vi "AB_900_1000_Project_RESTfulWebService_Info.vi"(7 "action":T2, 8 "error in (no error)":errorcluster, 10 "RESTfulWebServiceInfo in":T1, 11 "Object In":T3) -> (0 "error out":errorcluster, 2 "RESTfulWebServiceInfo out":T1, 3 "Object Out":T3)   [LabVIEW 2020]
uses:
  <resource>/Framework/Providers/API/ItemRef.ctl
  <vilib>/AppBuilder/RW_Project/AB_RW_Project_PropBag_Action.ctl
  <vilib>/AppBuilder/RW_Project/AB_RW_Project_RESTful_RoutingTemplate.ctl
  <vilib>/AppBuilder/AB_Classes/RESTful/AB_RESTful_RoutingType.ctl
  <vilib>/AppBuilder/AB_Classes/RESTful/AB_RESTful_HTTPMethodType.ctl
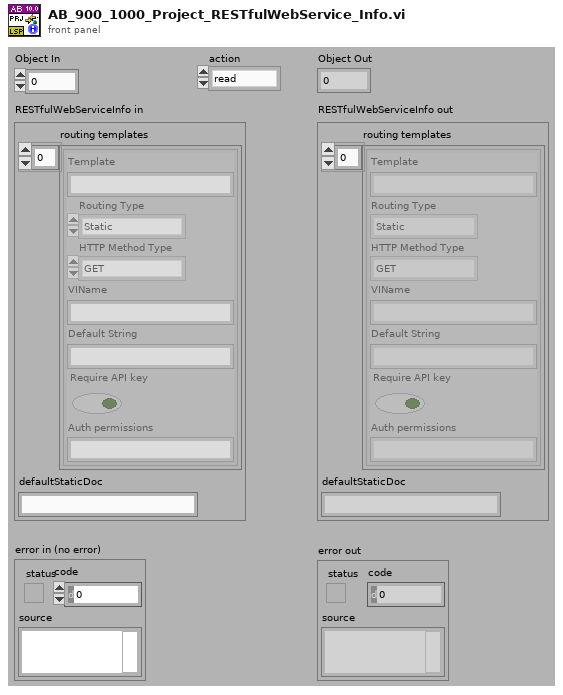
[diagram p1: front panel]
types:
  T1 = cluster{"routing templates":cluster{"Template":string, "Routing Type":enum32{"Method", "Static"}, "HTTP Method Type":enum32{"GET", "POST", "PUT", "DELETE"}, "VIName":string, "Default String":string, "Require API key":bool, "Auth permissions":string}[], "defaultStaticDoc":string}
  T2 = typedef "AB_RW_Project_PropBag_Action.ctl" = enum16{"read", "write", "clear", "readPrevious", "writePrevious", "clearPrevious"}
  T3 = typedef "ItemRef.ctl" = u64
  T4 = typedef "AB_RW_Project_RESTful_RoutingTemplate.ctl" = cluster{"Template":string, "Routing Type":T5, "HTTP Method Type":T6, "VIName":string, "Default String":string, "Require API key":bool, "Auth permissions":string}
  T5 = typedef "AB_RESTful_RoutingType.ctl" = enum32{"Method", "Static"}
  T6 = typedef "AB_RESTful_HTTPMethodType.ctl" = enum32{"GET", "POST", "PUT", "DELETE"}
  T7 = cluster{"Template":string, "Routing Type":enum32{"Method", "Static"}, "HTTP Method Type":enum32{"GET", "POST", "PUT", "DELETE"}, "VIName":string, "Default String":string, "Require API key":bool, "Auth permissions":string}[]
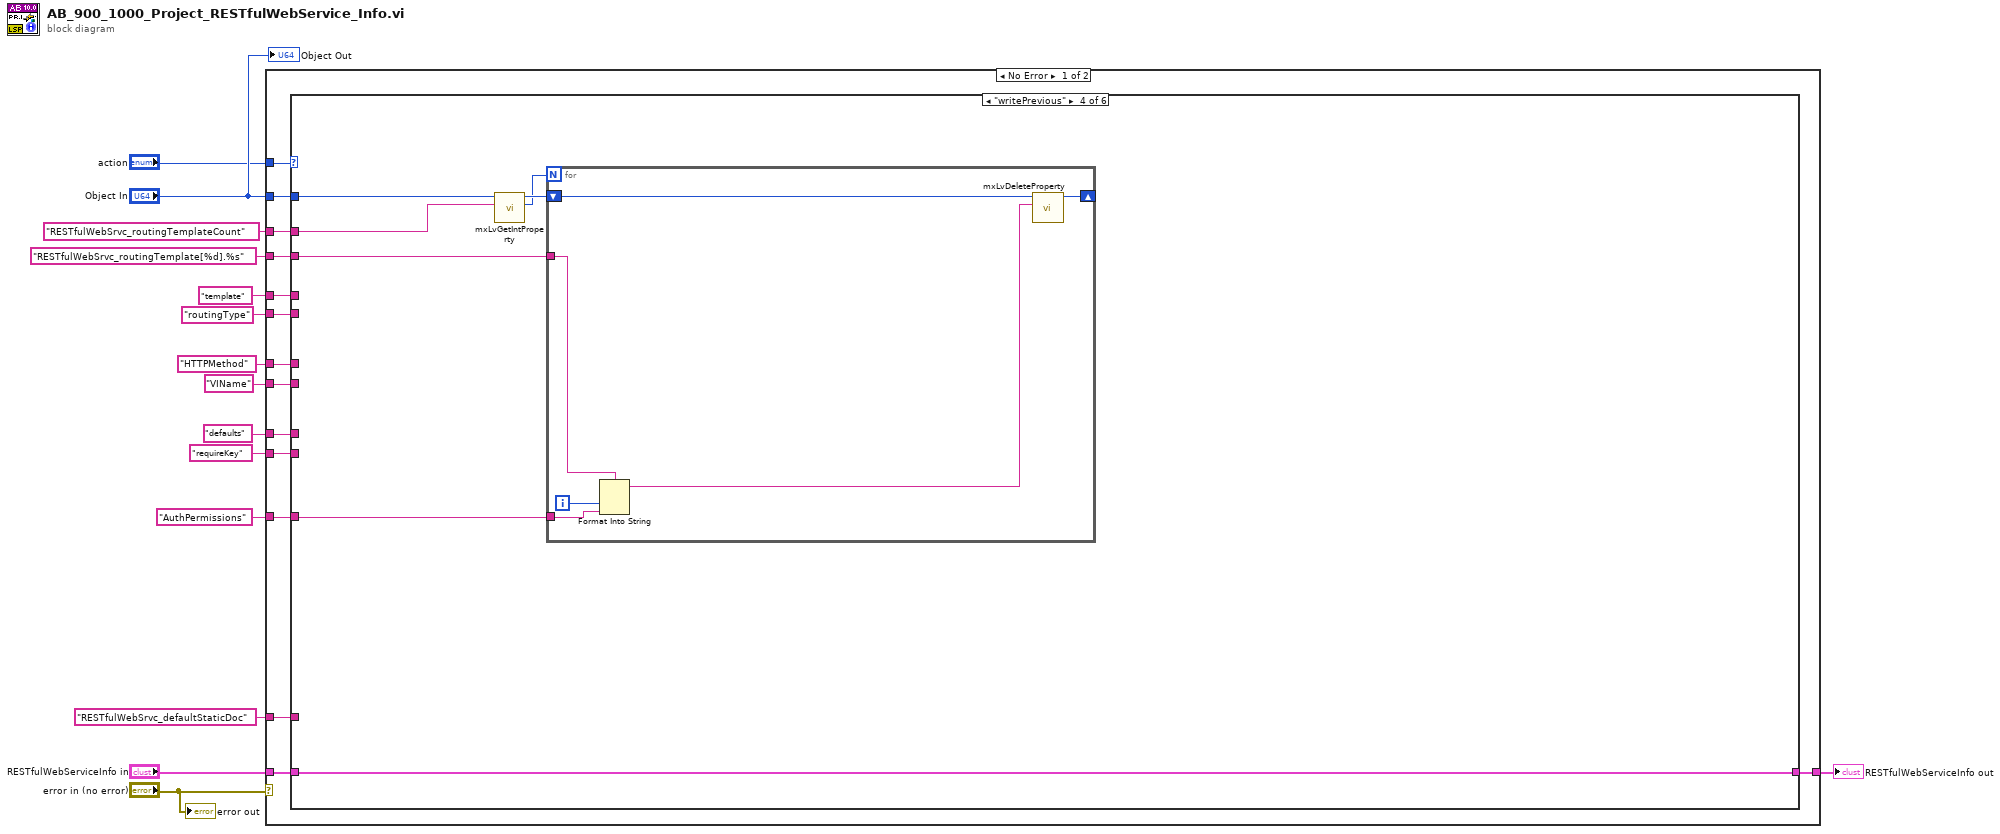
[diagram p0: block diagram]
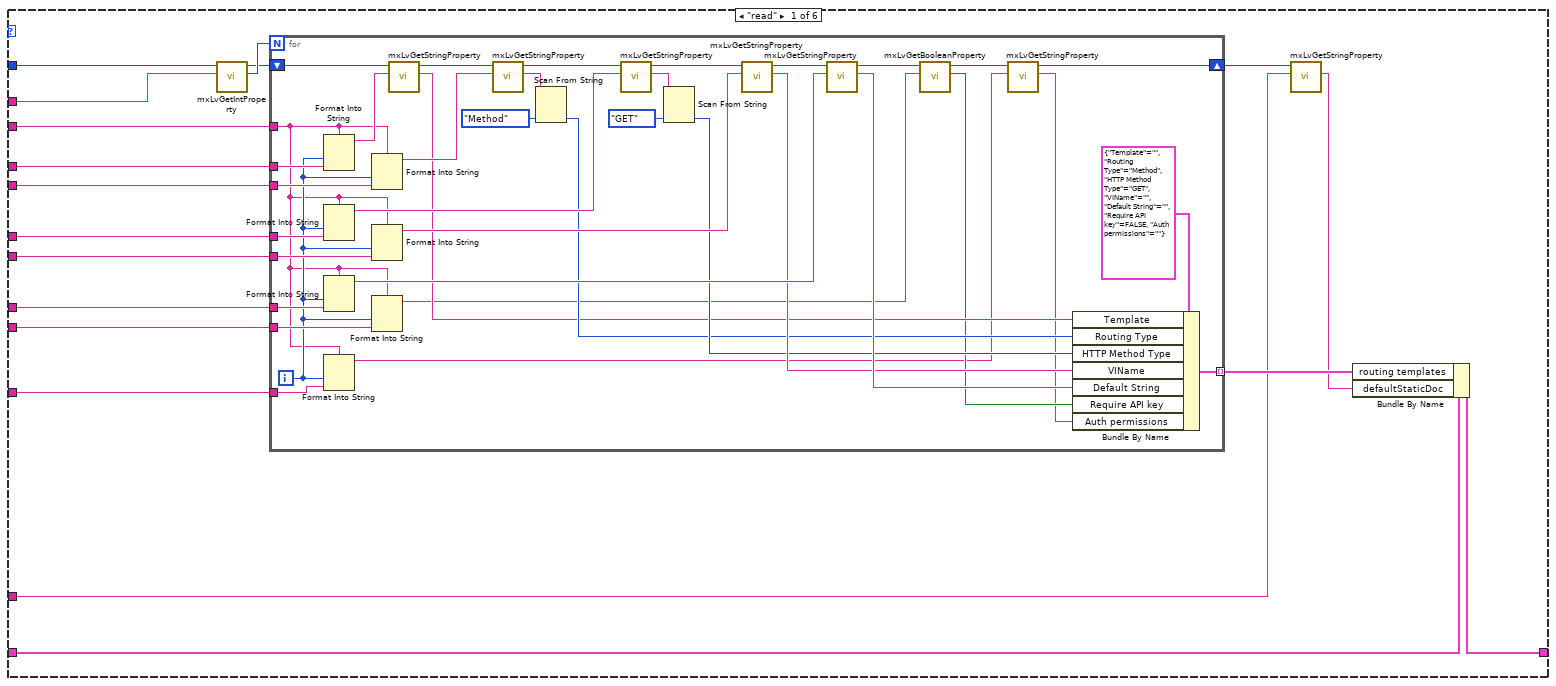
[diagram p2: hidden frame]
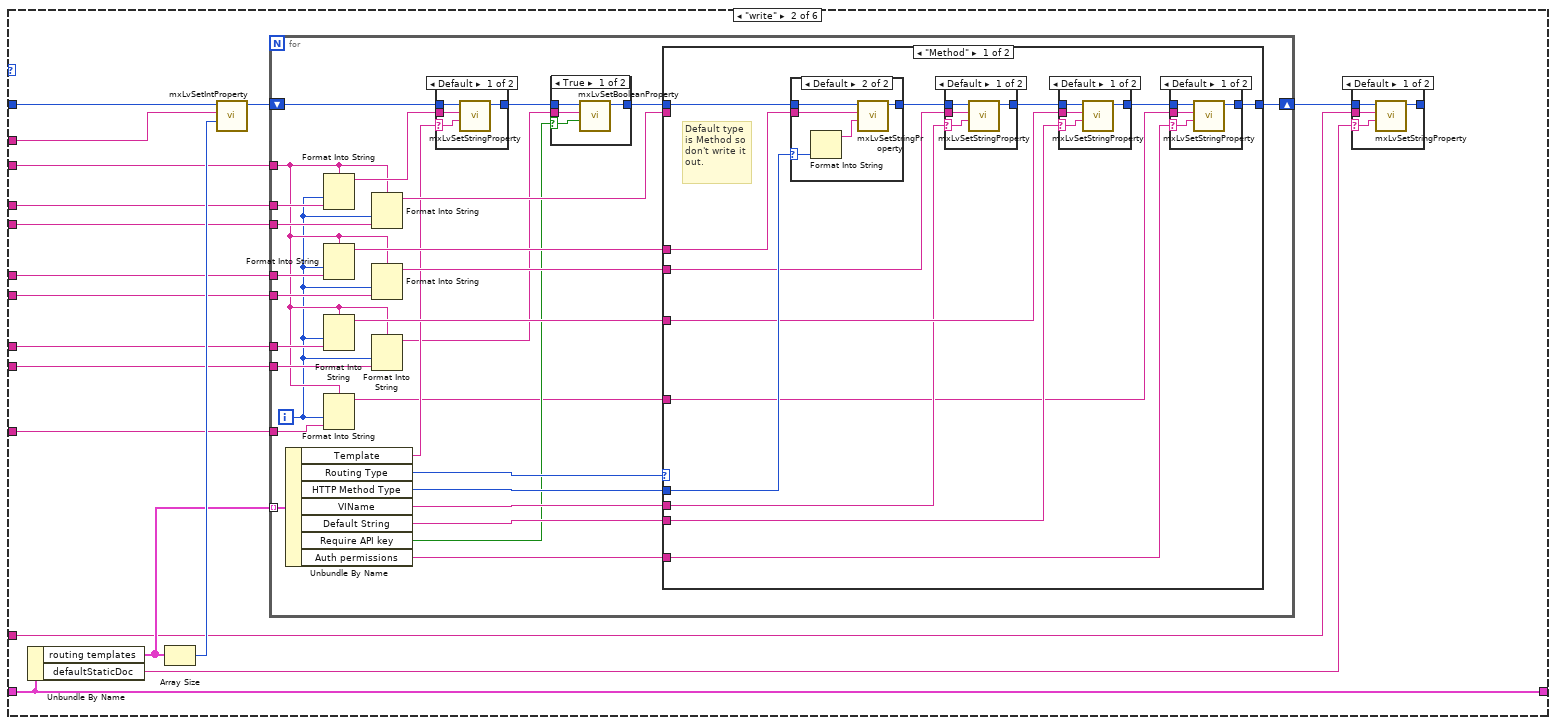
[diagram p3: hidden frame]
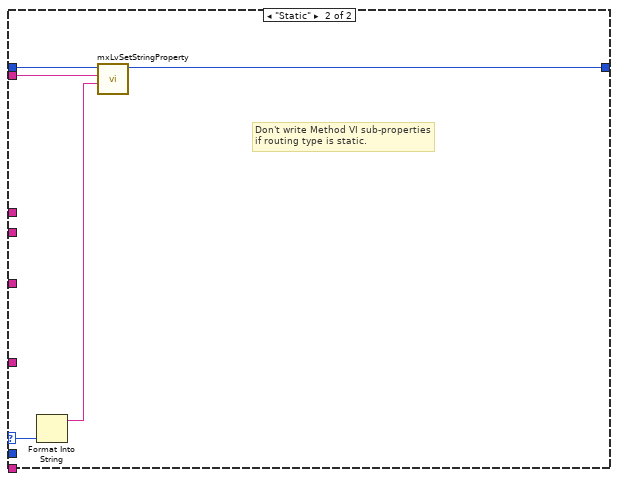
[diagram p10: hidden frame]
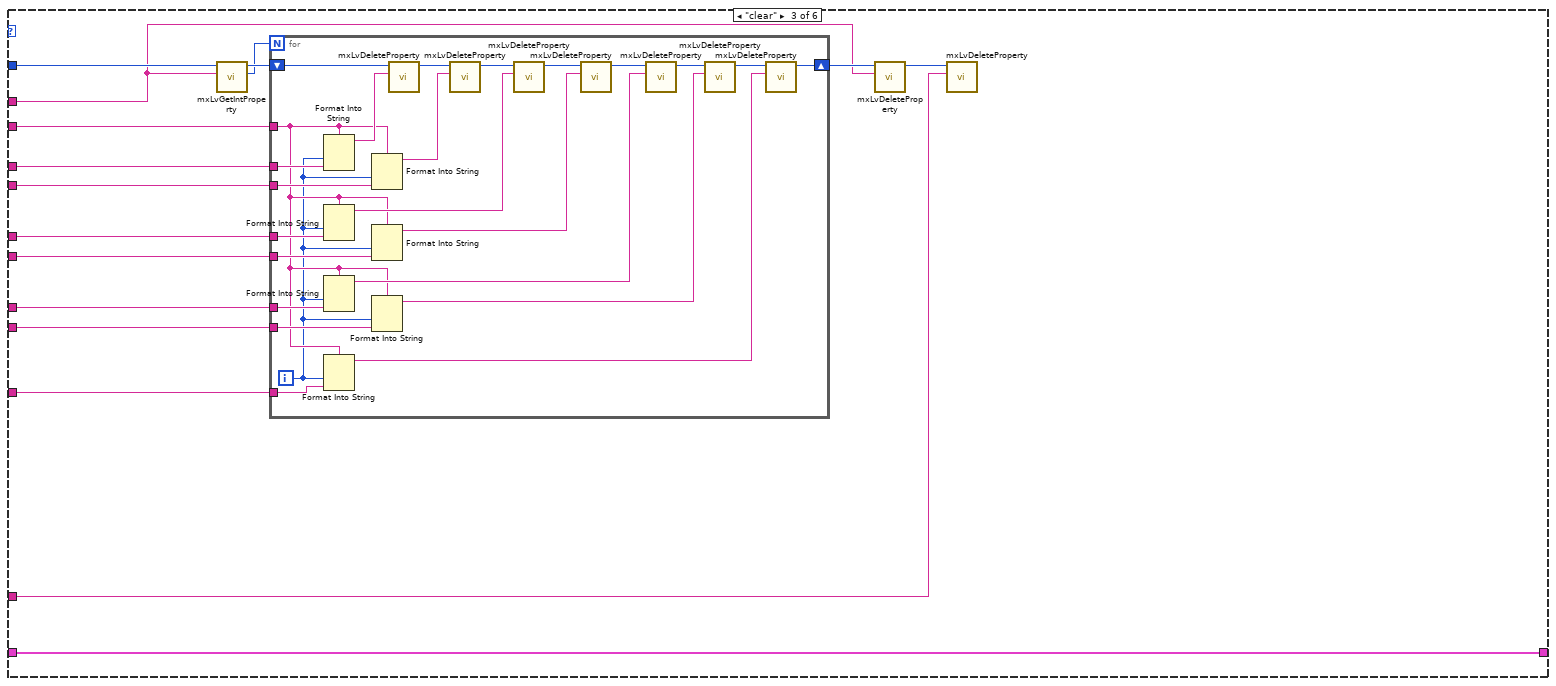
[diagram p12: hidden frame]
diagram:
  n1 = case shown="No Error" "error in (no error)" {
    tunnel: "Object In" -> [w29 _]
    tunnel: [w23 _] -> w8
    tunnel: "RESTfulWebSrvc_routingTemplateCount" ("Tag") -> [w28 _]
    tunnel: "RESTfulWebSrvc_routingTemplate[%d].%s" ("Tag") -> [w27 _]
    tunnel: "template" ("Tag") -> [w26 _]
    tunnel: "RESTfulWebServiceInfo in" -> [w25 _]
    tunnel: "action" -> [w24 _]
    tunnel: "routingType" ("Tag") -> [w22 _]
    tunnel: "HTTPMethod" ("Tag") -> [w21 _]
    tunnel: "VIName" ("Tag") -> [w20 _]
    tunnel: "defaults" ("Tag") -> [w19 _]
    tunnel: "requireKey" ("Tag") -> [w18 _]
    tunnel: "RESTfulWebSrvc_defaultStaticDoc" ("Tag") -> [w17 _]
    tunnel: "AuthPermissions" ("Tag") -> [w16 _]
    frame No Error {
      n2 = case shown="\"writePrevious\"" w24 {
        tunnel: w29 -> [w41 w98 w198 w229 _ _]
        tunnel: w28 -> [w47 w100 w189 w226 _ _]
        tunnel: w27 -> [w45 w96 w196 w227 _ _]
        tunnel: w26 -> [w40 w95 w195 _ _ _]
        tunnel: w25 -> [w42 w99 w197 w228 w237 w238]
        tunnel: [w43 w99 w197 w228 w237 w238] -> w23
        tunnel: w22 -> [w39 w94 w194 _ _ _]
        tunnel: w21 -> [w38 w93 w193 _ _ _]
        tunnel: w20 -> [w37 w92 w192 _ _ _]
        tunnel: w19 -> [w36 w91 w191 _ _ _]
        tunnel: w18 -> [w34 w89 w188 _ _ _]
        tunnel: w17 -> [w32 w87 w185 _ _ _]
        tunnel: w16 -> [w30 w85 w184 w224 _ _]
        frame "read" {
          n3 = call <resource>:"mxLvGetIntProperty.vi"("Tag"=w47, "Item"=w41) -> ("Value"=w46:i32, "Item"=w44:T3)  [unwired: 1 in, 7 out]
          n4 = for {
            N: w46 -> [_]
            shift-right: [w50] -> w33
            shift-left: w44 -> [w84]
            tunnel: w45 -> [w53]
            tunnel: w40 -> [w81]
            tunnel: w39 -> [w80]
            tunnel: w38 -> [w79]
            tunnel: w37 -> [w78]
            tunnel: w36 -> [w77]
            tunnel: [w60] -> w35 mode=indexing
            tunnel: w34 -> [w57]
            tunnel: w30 -> [w52]
            i -> [w54]
            n5 = Format Into String(format string=w53, w54, w81) -> (resulting string=w76:string)  [unwired: 2 in, 1 out]
            n6 = Format Into String(format string=w53, w54, w79) -> (resulting string=w71:string)  [unwired: 2 in, 1 out]
            n7 = Format Into String(format string=w53, w54, w77) -> (resulting string=w66:string)  [unwired: 2 in, 1 out]
            n8 = Format Into String(format string=w53, w54, w52) -> (resulting string=w48:string)  [unwired: 2 in, 1 out]
            n9 = Format Into String(format string=w53, w54, w80) -> (resulting string=w75:string)  [unwired: 2 in, 1 out]
            n10 = Format Into String(format string=w53, w54, w78) -> (resulting string=w67:string)  [unwired: 2 in, 1 out]
            n11 = Format Into String(format string=w53, w54, w57) -> (resulting string=w56:string)  [unwired: 2 in, 1 out]
            n12 = call <resource>:"mxLvGetStringProperty.vi"("Tag"=w76, "Item"=w84) -> ("Value"=w61:string, "Item"=w83:T3)  [unwired: 1 in, 7 out]
            n13 = call <resource>:"mxLvGetStringProperty.vi"("Tag"=w75, "Item"=w83) -> ("Value"=w82:string, "Item"=w72:T3)  [unwired: 1 in, 7 out]
            n14 = Scan From String(input string=w82, default 1=AB_RESTful_RoutingType."Method" ("Routing Type")) -> (output 1=w62:T5)  [unwired: 3 in, 3 out]
            n15 = call <resource>:"mxLvGetStringProperty.vi"("Tag"=w71, "Item"=w72) -> ("Value"=w73:string, "Item"=w68:T3)  [unwired: 1 in, 7 out]
            n16 = Scan From String(input string=w73, default 1=AB_RESTful_HTTPMethodType."GET" ("HTTP Method Type")) -> (output 1=w63:T6)  [unwired: 3 in, 3 out]
            n17 = call <resource>:"mxLvGetStringProperty.vi"("Tag"=w67, "Item"=w68) -> ("Value"=w64:string, "Item"=w69:T3)  [unwired: 1 in, 7 out]
            n18 = call <resource>:"mxLvGetStringProperty.vi"("Tag"=w66, "Item"=w69) -> ("Value"=w65:string, "Item"=w59:T3)  [unwired: 1 in, 7 out]
            n19 = call <resource>:"mxLvGetBooleanProperty.vi"("Tag"=w56, "Item"=w59) -> ("Value"=w58:bool, "Item"=w51:T3)  [unwired: 1 in, 7 out]
            n20 = call <resource>:"mxLvGetStringProperty.vi"("Tag"=w48, "Item"=w51) -> ("Value"=w49:string, "Item"=w50:T3)  [unwired: 1 in, 7 out]
            n21 = Bundle By Name(cluster=T4 {"Template"="", "Routing Type"=enum."Method", "HTTP Method Type"=enum."GET", "VIName"="", "Default String"="", "Require API key"=FALSE, "Auth permissions"=""} ("RESTful VI routing template"), "Template"=w61, "Routing Type"=w62, "HTTP Method Type"=w63, "VIName"=w64, "Default String"=w65, "Require API key"=w58, "Auth permissions"=w49) -> (w60:T4)
          }
          n22 = call <resource>:"mxLvGetStringProperty.vi"("Tag"=w32, "Item"=w33) -> ("Value"=w31:string)  [unwired: 1 in, 8 out]
          n23 = Bundle By Name(cluster=w42, "routing templates"=w35, "defaultStaticDoc"=w31) -> (w43:T1)
        }
        frame "write" {
          n24 = Unbundle By Name(w99) -> ("routing templates"=w90:T7, "defaultStaticDoc"=w86:string)
          n25 = Array Size(array=w90) -> (size(s)=w101:i32)
          n26 = call <resource>:"mxLvSetIntProperty.vi"("Value (0)"=w101, "Tag"=w100, "Item"=w98) -> ("Item"=w97:T3)  [unwired: 2 in, 6 out]
          n27 = for {
            shift-right: [w121] -> w88
            shift-left: w97 -> [w118]
            tunnel: w96 -> [w111]
            tunnel: w95 -> [w134]
            tunnel: w94 -> [w133]
            tunnel: w93 -> [w132]
            tunnel: w92 -> [w131]
            tunnel: w91 -> [w130]
            tunnel: w90 -> [w126] mode=indexing
            tunnel: w89 -> [w116]
            tunnel: w85 -> [w109]
            i -> [w110]
            n28 = Unbundle By Name(w126) -> ("Template"=w120:string, "Routing Type"=w117:enum32{"Method", "Static"}, "HTTP Method Type"=w125:enum32{"GET", "POST", "PUT", "DELETE"}, "VIName"=w124:string, "Default String"=w123:string, "Require API key"=w113:bool, "Auth permissions"=w107:string)
            n29 = Format Into String(format string=w111, w110, w134) -> (resulting string=w119:string)  [unwired: 2 in, 1 out]
            n30 = Format Into String(format string=w111, w110, w132) -> (resulting string=w128:string)  [unwired: 2 in, 1 out]
            n31 = Format Into String(format string=w111, w110, w130) -> (resulting string=w122:string)  [unwired: 2 in, 1 out]
            n32 = Format Into String(format string=w111, w110, w109) -> (resulting string=w108:string)  [unwired: 2 in, 1 out]
            n33 = Format Into String(format string=w111, w110, w133) -> (resulting string=w129:string)  [unwired: 2 in, 1 out]
            n34 = Format Into String(format string=w111, w110, w131) -> (resulting string=w127:string)  [unwired: 2 in, 1 out]
            n35 = Format Into String(format string=w111, w110, w116) -> (resulting string=w112:string)  [unwired: 2 in, 1 out]
            n36 = case shown="Default" w120 {
              selector: w120 -> [w179 _]
              tunnel: w118 -> [w182 w183]
              tunnel: w119 -> [w181 _]
              tunnel: [w180 w183] -> w115
              frame Default {
                n37 = call <resource>:"mxLvSetStringProperty.vi"("Value (\"\")"=w179, "Tag"=w181, "Item"=w182) -> ("Item"=w180:T3)  [unwired: 2 in, 6 out]
              }
              frame "" {
              }
            }
            n38 = case shown="True" w113 {
              selector: w113 -> [w137 _]
              tunnel: w115 -> [w138 w139]
              tunnel: w112 -> [w135 _]
              tunnel: [w136 w139] -> w114
              frame True {
                n39 = call <resource>:"mxLvSetBooleanProperty.vi"("Value (F)"=w137, "Tag"=w135, "Item"=w138) -> ("Item"=w136:T3)  [unwired: 2 in, 6 out]
              }
              frame False {
              }
            }
            n40 = case shown="\"Method\"" w117 {
              selector: w117 -> [_ w174]
              tunnel: w129 -> [_ w175]
              tunnel: w128 -> [w152 _]
              tunnel: w127 -> [w146 _]
              tunnel: w125 -> [w150 _]
              tunnel: w124 -> [w147 _]
              tunnel: w123 -> [w149 _]
              tunnel: w122 -> [w148 _]
              tunnel: [w142 w176] -> w121
              tunnel: w114 -> [w151 w177]
              tunnel: w108 -> [w141 _]
              tunnel: w107 -> [w140 _]
              frame "Method" {
                # "Default type is Method so don't write it out."
                n41 = case shown="Default" w150 {
                  selector: w150 -> [_ w169]
                  tunnel: w152 -> [_ w173]
                  tunnel: [w168 w172] -> w145
                  tunnel: w151 -> [w168 w170]
                  frame "GET" {
                    # "Don't write out default."
                  }
                  frame Default {
                    n42 = Format Into String(w169) -> (resulting string=w171:string)  [unwired: 3 in, 1 out]
                    n43 = call <resource>:"mxLvSetStringProperty.vi"("Value (\"\")"=w171, "Tag"=w173, "Item"=w170) -> ("Item"=w172:T3)  [unwired: 2 in, 6 out]
                  }
                }
                n44 = case shown="Default" w147 {
                  selector: w147 -> [w158 _]
                  tunnel: w145 -> [w161 w162]
                  tunnel: w146 -> [w160 _]
                  tunnel: [w159 w162] -> w144
                  frame Default {
                    n45 = call <resource>:"mxLvSetStringProperty.vi"("Value (\"\")"=w158, "Tag"=w160, "Item"=w161) -> ("Item"=w159:T3)  [unwired: 2 in, 6 out]
                  }
                  frame "" {
                  }
                }
                n46 = case shown="Default" w149 {
                  selector: w149 -> [w163 _]
                  tunnel: w144 -> [w166 w167]
                  tunnel: w148 -> [w165 _]
                  tunnel: [w164 w167] -> w143
                  frame Default {
                    n47 = call <resource>:"mxLvSetStringProperty.vi"("Value (\"\")"=w163, "Tag"=w165, "Item"=w166) -> ("Item"=w164:T3)  [unwired: 2 in, 6 out]
                  }
                  frame "" {
                  }
                }
                n48 = case shown="Default" w140 {
                  selector: w140 -> [w153 _]
                  tunnel: w143 -> [w156 w157]
                  tunnel: w141 -> [w155 _]
                  tunnel: [w154 w157] -> w142
                  frame Default {
                    n49 = call <resource>:"mxLvSetStringProperty.vi"("Value (\"\")"=w153, "Tag"=w155, "Item"=w156) -> ("Item"=w154:T3)  [unwired: 2 in, 6 out]
                  }
                  frame "" {
                  }
                }
              }
              frame "Static" {
                # "Don't write Method VI sub-properties if routing type is static."
                n50 = Format Into String(w174) -> (resulting string=w178:string)  [unwired: 3 in, 1 out]
                n51 = call <resource>:"mxLvSetStringProperty.vi"("Value (\"\")"=w178, "Tag"=w175, "Item"=w177) -> ("Item"=w176:T3)  [unwired: 2 in, 6 out]
              }
            }
          }
          n52 = case shown="Default" w86 {
            selector: w86 -> [w102 _]
            tunnel: w88 -> [w105 w106]
            tunnel: w87 -> [w104 _]
            tunnel: [w103 w106] -> _
            frame Default {
              n53 = call <resource>:"mxLvSetStringProperty.vi"("Value (\"\")"=w102, "Tag"=w104, "Item"=w105) -> ("Item"=w103:T3)  [unwired: 2 in, 6 out]
            }
            frame "" {
            }
          }
        }
        frame "clear" {
          n54 = call <resource>:"mxLvGetIntProperty.vi"("Tag"=w189, "Item"=w198) -> ("Value"=w187:i32, "Item"=w199:T3)  [unwired: 1 in, 7 out]
          n55 = for {
            N: w187 -> [_]
            shift-right: [w201] -> w190
            shift-left: w199 -> [w223]
            tunnel: w196 -> [w205]
            tunnel: w195 -> [w221]
            tunnel: w194 -> [w220]
            tunnel: w193 -> [w219]
            tunnel: w192 -> [w218]
            tunnel: w191 -> [w217]
            tunnel: w188 -> [w206]
            tunnel: w184 -> [w203]
            i -> [w204]
            n56 = Format Into String(format string=w205, w204, w221) -> (resulting string=w216:string)  [unwired: 2 in, 1 out]
            n57 = Format Into String(format string=w205, w204, w219) -> (resulting string=w213:string)  [unwired: 2 in, 1 out]
            n58 = Format Into String(format string=w205, w204, w217) -> (resulting string=w209:string)  [unwired: 2 in, 1 out]
            n59 = Format Into String(format string=w205, w204, w203) -> (resulting string=w200:string)  [unwired: 2 in, 1 out]
            n60 = Format Into String(format string=w205, w204, w220) -> (resulting string=w215:string)  [unwired: 2 in, 1 out]
            n61 = Format Into String(format string=w205, w204, w218) -> (resulting string=w210:string)  [unwired: 2 in, 1 out]
            n62 = Format Into String(format string=w205, w204, w206) -> (resulting string=w207:string)  [unwired: 2 in, 1 out]
            n63 = call <resource>:"mxLvDeleteProperty.vi"("Tag"=w216, "Item"=w223) -> ("Item"=w222:T3)  [unwired: 1 in, 8 out]
            n64 = call <resource>:"mxLvDeleteProperty.vi"("Tag"=w215, "Item"=w222) -> ("Item"=w214:T3)  [unwired: 1 in, 8 out]
            n65 = call <resource>:"mxLvDeleteProperty.vi"("Tag"=w213, "Item"=w214) -> ("Item"=w211:T3)  [unwired: 1 in, 8 out]
            n66 = call <resource>:"mxLvDeleteProperty.vi"("Tag"=w210, "Item"=w211) -> ("Item"=w212:T3)  [unwired: 1 in, 8 out]
            n67 = call <resource>:"mxLvDeleteProperty.vi"("Tag"=w209, "Item"=w212) -> ("Item"=w208:T3)  [unwired: 1 in, 8 out]
            n68 = call <resource>:"mxLvDeleteProperty.vi"("Tag"=w207, "Item"=w208) -> ("Item"=w202:T3)  [unwired: 1 in, 8 out]
            n69 = call <resource>:"mxLvDeleteProperty.vi"("Tag"=w200, "Item"=w202) -> ("Item"=w201:T3)  [unwired: 1 in, 8 out]
          }
          n70 = call <resource>:"mxLvDeleteProperty.vi"("Tag"=w189, "Item"=w190) -> ("Item"=w186:T3)  [unwired: 1 in, 8 out]
          n71 = call <resource>:"mxLvDeleteProperty.vi"("Tag"=w185, "Item"=w186) -> ()  [unwired: 1 in, 9 out]
        }
        frame "writePrevious" {
          n72 = call <resource>:"mxLvGetIntProperty.vi"("Tag"=w226, "Item"=w229) -> ("Value"=w225:i32, "Item"=w230:T3)  [unwired: 1 in, 7 out]
          n73 = for {
            N: w225 -> [_]
            shift-right: [w233] -> _
            shift-left: w230 -> [w231]
            tunnel: w227 -> [w236]
            tunnel: w224 -> [w234]
            i -> [w235]
            n74 = Format Into String(format string=w236, w235, w234) -> (resulting string=w232:string)  [unwired: 2 in, 1 out]
            n75 = call <resource>:"mxLvDeleteProperty.vi"("Tag"=w232, "Item"=w231) -> ("Item"=w233:T3)  [unwired: 1 in, 8 out]
          }
        }
        frame "readPrevious" {
        }
        frame "clearPrevious" {
        }
      }
    }
    frame Error {
    }
  }
  "RESTfulWebServiceInfo out" <- w8
  "Object Out" <- "Object In"
  "error out" <- "error in (no error)"
